vi "Save Config.vi"(10 "Cluster":T1, 11 "Process":bool) -> ()   [LabVIEW 2016]
uses:
  <vilib>/Utility/config.llb/Write Key (Double).vi
  <vilib>/Utility/config.llb/Write Key (Boolean).vi
  <vilib>/Utility/config.llb/NI_LVConfig.lvlib
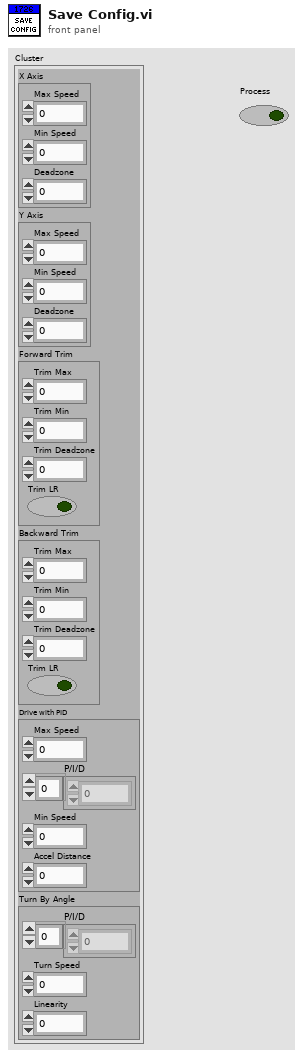
[diagram p1: front panel]
types:
  T1 = cluster{"X Axis":cluster{"Max Speed":dbl, "Min Speed":dbl, "Deadzone":dbl}, "Y Axis":cluster{"Max Speed":dbl, "Min Speed":dbl, "Deadzone":dbl}, "Forward Trim":cluster{"Trim Max":dbl, "Trim Min":dbl, "Trim Deadzone":dbl, "Trim LR":bool}, "Backward Trim":cluster{"Trim Max":dbl, "Trim Min":dbl, "Trim Deadzone":dbl, "Trim LR":bool}, "Drive with PID":cluster{"Max Speed":dbl, "P/I/D":dbl[], "Min Speed":dbl, "Accel Distance":dbl}, "Turn By Angle":cluster{"P/I/D":dbl[], "Turn Speed":dbl, "Linearity":dbl}}
  T2 = cluster{"Max Speed":dbl, "Min Speed":dbl, "Deadzone":dbl}
  T3 = cluster{"Trim Max":dbl, "Trim Min":dbl, "Trim Deadzone":dbl, "Trim LR":bool}
  T4 = cluster{"Max Speed":dbl, "P/I/D":dbl[], "Min Speed":dbl, "Accel Distance":dbl}
  T5 = cluster{"P/I/D":dbl[], "Turn Speed":dbl, "Linearity":dbl}
  T6 = typedef "NI_LVConfig.lvlib/Config Data RefNum.ctl" = refnum<k1>
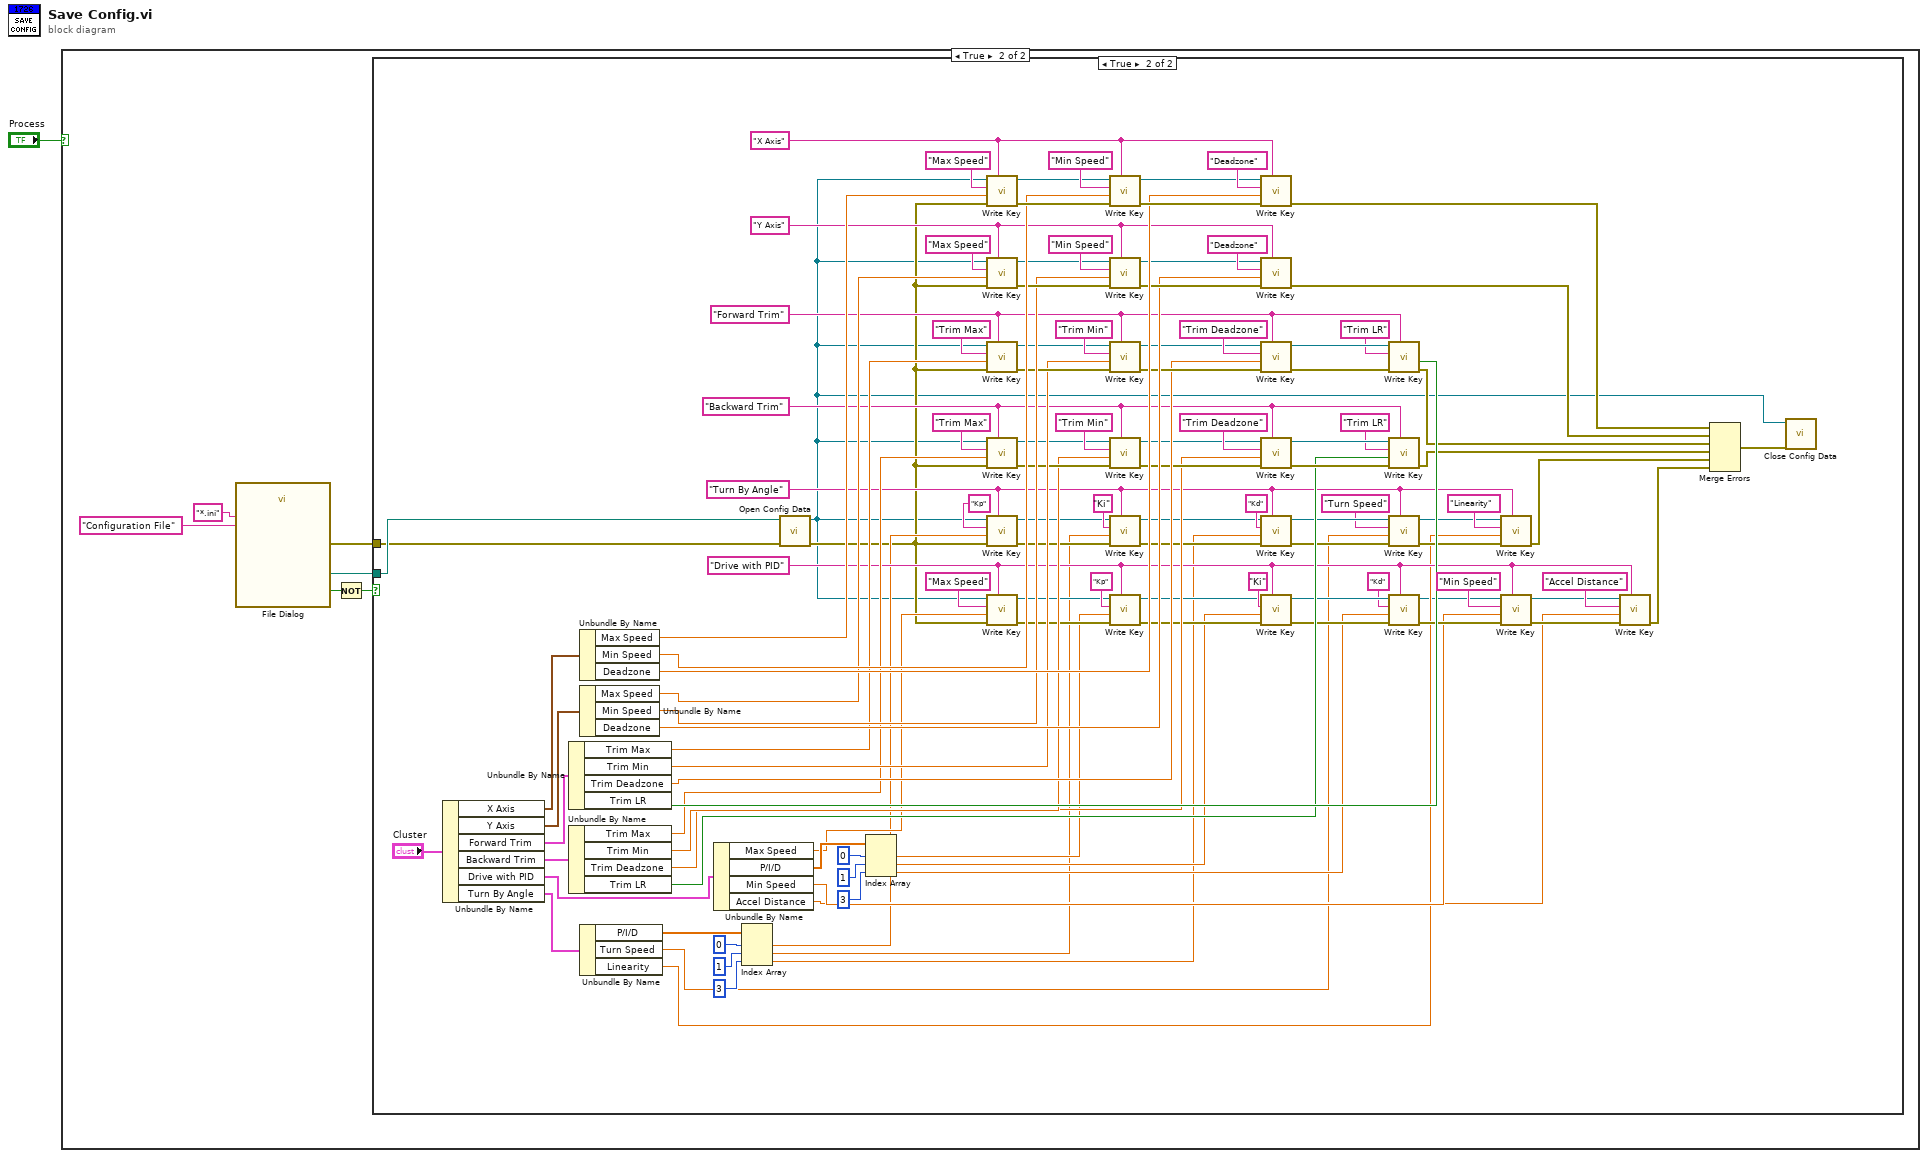
[diagram p0: block diagram]
diagram:
  n1 = case shown="True" "Process" {
    frame False {
    }
    frame True {
      n2 = call "File Dialog"("pattern (all files)"="*.ini", "pattern label"="Configuration File") -> ("selected path"=w3:path, "cancelled"=w5:bool, "error out"=w2:errorcluster)  [unwired: 10 in, 1 out]
      n3 = Not(x=w5) -> (.not. x?=w4:bool)
      n4 = case shown="True" w4 {
        tunnel: w3 -> [_ w112]
        tunnel: w2 -> [_ w111]
        frame False {
        }
        frame True {
          w25 = "Turn By Angle" ("section")
          w44 = "Drive with PID" ("section")
          w63 = "Backward Trim" ("section")
          w83 = "Forward Trim" ("section")
          w99 = "Y Axis" ("section")
          w110 = "X Axis" ("section")
          n5 = Unbundle By Name("Cluster") -> ("X Axis"=w126:T2, "Y Axis"=w125:T2, "Forward Trim"=w124:T3, "Backward Trim"=w123:T3, "Drive with PID"=w122:T4, "Turn By Angle"=w121:T5)
          n6 = Unbundle By Name(w124) -> ("Trim Max"=w79:dbl, "Trim Min"=w78:dbl, "Trim Deadzone"=w75:dbl, "Trim LR"=w74:bool)
          n7 = Unbundle By Name(w123) -> ("Trim Max"=w62:dbl, "Trim Min"=w61:dbl, "Trim Deadzone"=w60:dbl, "Trim LR"=w59:bool)
          n8 = Unbundle By Name(w126) -> ("Max Speed"=w102:dbl, "Min Speed"=w101:dbl, "Deadzone"=w100:dbl)
          n9 = Unbundle By Name(w125) -> ("Max Speed"=w92:dbl, "Min Speed"=w91:dbl, "Deadzone"=w90:dbl)
          n10 = Unbundle By Name(w121) -> ("P/I/D"=w113:dbl[], "Turn Speed"=w21:dbl, "Linearity"=w20:dbl)
          n11 = Unbundle By Name(w122) -> ("Max Speed"=w43:dbl, "P/I/D"=w120:dbl[], "Min Speed"=w39:dbl, "Accel Distance"=w38:dbl)
          n12 = Index Array(array=w113, index #1=0 ("index"), index #2=1 ("index"), index #3=3 ("index")) -> (element #1=w24:dbl, element #2=w23:dbl, element #3=w22:dbl)
          n13 = call <vilib>:"Open Config Data.vi"("error in (no error)"=w111, "configuration file path"=w112) -> ("error out"=w19:errorcluster, "refnum"=w10:T6)  [unwired: 7 in, 1 out]
          n14 = Index Array(array=w120, index #1=0 ("index"), index #2=1 ("index"), index #3=3 ("index")) -> (element #1=w42:dbl, element #2=w41:dbl, element #3=w40:dbl)
          n15 = call-poly <vilib>:"Write Key.vi"("section"=w110, "error in (no error)"=w19, "value"=w102, "key"="Max Speed", "refnum"=w10) -> ("error out"=w109:errorcluster, "refnum out"=w104:T6)  [unwired: 4 in, 1 out]
          n16 = call-poly <vilib>:"Write Key.vi"("section"=w99, "error in (no error)"=w19, "value"=w92, "key"="Max Speed", "refnum"=w10) -> ("error out"=w98:errorcluster, "refnum out"=w94:T6)  [unwired: 4 in, 1 out]
          n17 = call-poly <vilib>:"Write Key.vi"("section"=w83, "error in (no error)"=w19, "value"=w79, "key"="Trim Max", "refnum"=w10) -> ("error out"=w89:errorcluster, "refnum out"=w85:T6)  [unwired: 4 in, 1 out]
          n18 = call-poly <vilib>:"Write Key.vi"("section"=w63, "error in (no error)"=w19, "value"=w62, "key"="Trim Max", "refnum"=w10) -> ("error out"=w73:errorcluster, "refnum out"=w69:T6)  [unwired: 4 in, 1 out]
          n19 = call-poly <vilib>:"Write Key.vi"("section"=w25, "error in (no error)"=w19, "value"=w24, "key"="Kp", "refnum"=w10) -> ("error out"=w37:errorcluster, "refnum out"=w33:T6)  [unwired: 4 in, 1 out]
          n20 = call-poly <vilib>:"Write Key.vi"("section"=w44, "error in (no error)"=w19, "value"=w43, "key"="Max Speed", "refnum"=w10) -> ("error out"=w58:errorcluster, "refnum out"=w54:T6)  [unwired: 4 in, 1 out]
          n21 = call-poly <vilib>:"Write Key.vi"("section"=w110, "error in (no error)"=w109, "value"=w101, "key"="Min Speed", "refnum"=w104) -> ("error out"=w108:errorcluster, "refnum out"=w103:T6)  [unwired: 4 in, 1 out]
          n22 = call-poly <vilib>:"Write Key.vi"("section"=w99, "error in (no error)"=w98, "value"=w91, "key"="Min Speed", "refnum"=w94) -> ("error out"=w97:errorcluster, "refnum out"=w93:T6)  [unwired: 4 in, 1 out]
          n23 = call-poly <vilib>:"Write Key.vi"("section"=w83, "error in (no error)"=w89, "value"=w78, "key"="Trim Min", "refnum"=w85) -> ("error out"=w88:errorcluster, "refnum out"=w84:T6)  [unwired: 4 in, 1 out]
          n24 = call-poly <vilib>:"Write Key.vi"("section"=w63, "error in (no error)"=w73, "value"=w61, "key"="Trim Min", "refnum"=w69) -> ("error out"=w72:errorcluster, "refnum out"=w68:T6)  [unwired: 4 in, 1 out]
          n25 = call-poly <vilib>:"Write Key.vi"("section"=w25, "error in (no error)"=w37, "value"=w23, "key"="Ki", "refnum"=w33) -> ("error out"=w36:errorcluster, "refnum out"=w32:T6)  [unwired: 4 in, 1 out]
          n26 = call-poly <vilib>:"Write Key.vi"("section"=w44, "error in (no error)"=w58, "value"=w42, "key"="Kp", "refnum"=w54) -> ("error out"=w57:errorcluster, "refnum out"=w53:T6)  [unwired: 4 in, 1 out]
          n27 = call-poly <vilib>:"Write Key.vi"("section"=w110, "error in (no error)"=w108, "value"=w100, "key"="Deadzone", "refnum"=w103) -> ("error out"=w15:errorcluster)  [unwired: 4 in, 2 out]
          n28 = call-poly <vilib>:"Write Key.vi"("section"=w99, "error in (no error)"=w97, "value"=w90, "key"="Deadzone", "refnum"=w93) -> ("error out"=w14:errorcluster)  [unwired: 4 in, 2 out]
          n29 = call-poly <vilib>:"Write Key.vi"("section"=w83, "error in (no error)"=w88, "value"=w75, "key"="Trim Deadzone", "refnum"=w84) -> ("error out"=w82:errorcluster, "refnum out"=w81:T6)  [unwired: 4 in, 1 out]
          n30 = call-poly <vilib>:"Write Key.vi"("section"=w63, "error in (no error)"=w72, "value"=w60, "key"="Trim Deadzone", "refnum"=w68) -> ("error out"=w67:errorcluster, "refnum out"=w66:T6)  [unwired: 4 in, 1 out]
          n31 = call-poly <vilib>:"Write Key.vi"("section"=w25, "error in (no error)"=w36, "value"=w22, "key"="Kd", "refnum"=w32) -> ("error out"=w31:errorcluster, "refnum out"=w30:T6)  [unwired: 4 in, 1 out]
          n32 = call-poly <vilib>:"Write Key.vi"("section"=w44, "error in (no error)"=w57, "value"=w41, "key"="Ki", "refnum"=w53) -> ("error out"=w52:errorcluster, "refnum out"=w51:T6)  [unwired: 4 in, 1 out]
          n33 = call-poly <vilib>:"Write Key.vi"("section"=w83, "error in (no error)"=w82, "value"=w74, "key"="Trim LR", "refnum"=w81) -> ("error out"=w13:errorcluster)  [unwired: 4 in, 2 out]
          n34 = call-poly <vilib>:"Write Key.vi"("section"=w63, "error in (no error)"=w67, "value"=w59, "key"="Trim LR", "refnum"=w66) -> ("error out"=w12:errorcluster)  [unwired: 4 in, 2 out]
          n35 = call-poly <vilib>:"Write Key.vi"("section"=w25, "error in (no error)"=w31, "value"=w21, "key"="Turn Speed", "refnum"=w30) -> ("error out"=w26:errorcluster, "refnum out"=w18:T6)  [unwired: 4 in, 1 out]
          n36 = call-poly <vilib>:"Write Key.vi"("section"=w44, "error in (no error)"=w52, "value"=w40, "key"="Kd", "refnum"=w51) -> ("error out"=w46:errorcluster, "refnum out"=w17:T6)  [unwired: 4 in, 1 out]
          n37 = call-poly <vilib>:"Write Key.vi"("section"=w25, "error in (no error)"=w26, "value"=w20, "key"="Linearity", "refnum"=w18) -> ("error out"=w9:errorcluster)  [unwired: 4 in, 2 out]
          n38 = call-poly <vilib>:"Write Key.vi"("section"=w44, "error in (no error)"=w46, "value"=w39, "key"="Min Speed", "refnum"=w17) -> ("error out"=w45:errorcluster, "refnum out"=w16:T6)  [unwired: 4 in, 1 out]
          n39 = call-poly <vilib>:"Write Key.vi"("section"=w44, "error in (no error)"=w45, "value"=w38, "key"="Accel Distance", "refnum"=w16) -> ("error out"=w8:errorcluster)  [unwired: 4 in, 2 out]
          n40 = Merge Errors(w15, w14, w13, w12, w9, w8) -> (w11:errorcluster)
          n41 = call <vilib>:"Close Config Data.vi"("error in (no error)"=w11, "refnum"=w10) -> ()  [unwired: 8 in, 2 out]
        }
      }
    }
  }
